vi "Configure Trigger.vi"(6 "Sample Interval (-1s)":dbl=-1.0 format="%.2f", 7 "Trigger Type Index":u16 caption="Trigger Type Index(0)", 8 "error in (no error)":errorcluster, 9 "Samples per Trigger":i32=1 caption="Samples per Trigger(1)", 10 "Triggers to measure":i32=1 caption="Triggers to measure(1)", 11 "NI DMM Driver in":refnum<class "DMM.NI.lvclass">) -> (0 "error dub":errorcluster, 1 "Success?":bool, 3 "NI DMM Driver out":refnum<class "DMM.NI.lvclass">)   [LabVIEW 2020, in "NI DMM Driver.lvlib" / "DMM.NI.lvclass"]
doc: "Configure the DMM for a triggered measurement."
uses:
  DMM.NI.lvclass
  <instrlib>/niDMM/nidmm.llb/niDMM Sample Trigger.ctl
  Controls/Ctl_MultiReadConfig.ctl
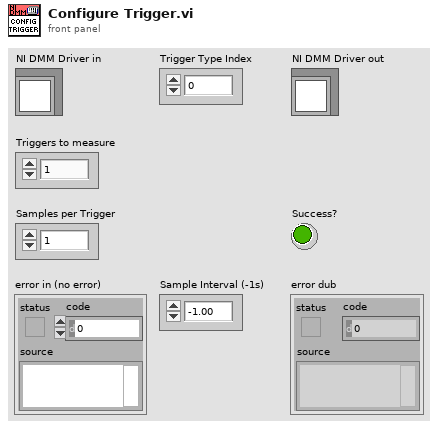
[diagram p1: front panel]
types:
  T1 = typedef "NI DMM Driver.lvlib/Ctl_MultiReadConfig.ctl" = cluster{"Trigger Count":i32, "Sample Count":i32, "Sample Trigger":T2, "Sample Interval (sec)":dbl}
  T2 = typedef "niDMM Sample Trigger.ctl" = enum16{"Immediate", "External", "TTL 0", "TTL 1", "TTL 2", "TTL 3", "TTL 4", "TTL 5", "TTL 6", "Interval", "Software", "TTL 7", "PXI Star", "LBR Trig 1", "Aux Trig 1"}
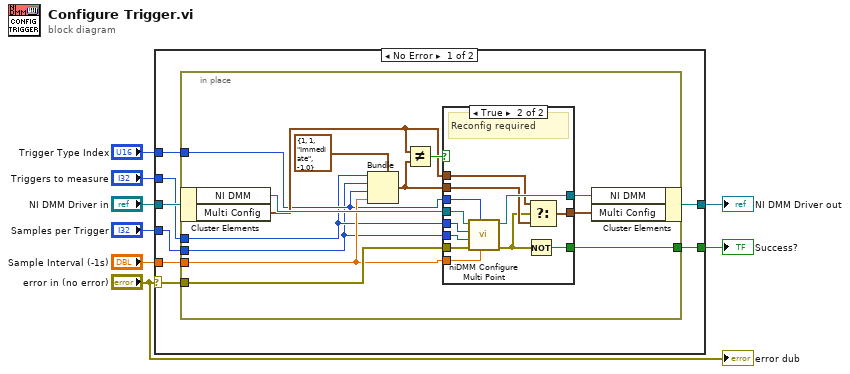
[diagram p0: block diagram]
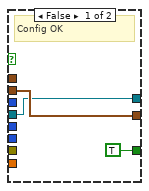
[diagram p2: hidden frame]
diagram:
  n1 = case shown="No Error" "error in (no error)" {
    selector: "error in (no error)" -> [w10 _]
    tunnel: [w9 w45] -> w8
    tunnel: "NI DMM Driver in" -> [w16 w45]
    tunnel: "Triggers to measure" -> [w15 _]
    tunnel: "Samples per Trigger" -> [w14 _]
    tunnel: "Sample Interval (-1s)" -> [w13 _]
    tunnel: "Trigger Type Index" -> [w12 _]
    tunnel: [w11 _] -> w2
    frame No Error {
      n2 = in-place {
        in-place-border: w15 -> [w18]
        in-place-border: w14 -> [w17]
        in-place-border: w13 -> [w20]
        in-place-border: w12 -> [w19]
        in-place-border: [w22] -> w11
        in-place-border: w10 -> [w21]
        n3 = in-place-cluster #1(w16) -> ("NI DMM"=w29:refnum<k15>, "Multi Config"=w24:T1)
        n4 = Bundle(cluster=T1 {"Trigger Count"=1, "Sample Count"=1, "Sample Trigger"=enum."Immediate", "Sample Interval (sec)"=-1.0} ("Multi Measure"), "Trigger Count"=w18, "Sample Count"=w17, "Sample Trigger"=w19, "Sample Interval (sec)"=w20) -> (w25:T1)
        n5 = Not Equal?(x=w24, y=w25) -> (x != y?=w26:bool)
        n6 = case shown="True" w26 {
          tunnel: w29 -> [w30 w44]
          tunnel: [w30 w43] -> w28
          tunnel: w25 -> [w31 w41]
          tunnel: w24 -> [_ w42]
          tunnel: [w31 w40] -> w23
          tunnel: [TRUE w38] -> w22
          tunnel: w21 -> [_ w33]
          tunnel: w20 -> [_ w37]
          tunnel: w19 -> [_ w36]
          tunnel: w18 -> [_ w35]
          tunnel: w17 -> [_ w34]
          frame False {
            # "Config OK"
          }
          frame True {
            # "Reconfig required"
            n7 = call <instrlib>:"niDMM Configure Multi Point.vi"("Sample Interval (sec)"=w37, "Sample Trigger"=w36, "error in (no error)"=w33, "Sample Count"=w34, "Trigger Count"=w35, "instrument handle"=w44) -> ("error out"=w39:errorcluster, "instrument handle out"=w43:refnum<k15>)  [unwired: 4 in]
            n8 = Not(x=w39) -> (.not. x?=w38:bool)
            n9 = Select(t=w42, s=w39, f=w41) -> (s? t:f=w40:T1)
          }
        }
        n10 = in-place-cluster #1("NI DMM"=w28, "Multi Config"=w23) -> (w9:refnum<class "DMM.NI.lvclass">)
      }
    }
    frame Error {
    }
  }
  "NI DMM Driver out" <- w8
  "Success?" <- w2
  "error dub" <- "error in (no error)"
